vi "cDAQ DDS Set.vi"(5 "common f [Hz]":dbl=1000.0, 6 "ofs [V]":dbl[](array[numeric]), 7 "f [Hz] (empty)":dbl[](array[numeric]), 8 "error in":errorcluster, 9 "ph [rad]":dbl[](array[numeric]), 10 "A [V]":dbl[](array[numeric]), 11 "cDAQ dds":T1={"device"="", "channels"=[], "mclk source"="", "mclk [Hz]"=0.0, "fs [Hz]"=0.0, "block [s]"=0.0, "buf [s]"=0.0, "task"="", "cmd queue"=refnum, "proc ref"=refnum, "smpl clock out"="/cDAQ3/PFI0", "export smpl clock"=FALSE, "DC ofs [V]"=[], "timebase source"="", "timebase mode"=enum."Local", "dither"=enum."Disabled", "dither level"=0.0} {"channels" min=0 step=1}) -> (0 "error out":errorcluster, 3 "cDAQ dds out":T1={"device"="", "channels"=[], "mclk source"="", "mclk [Hz]"=0.0, "fs [Hz]"=0.0, "block [s]"=0.0, "buf [s]"=0.0, "task"="", "cmd queue"=refnum, "proc ref"=refnum, "smpl clock out"="/cDAQ3/PFI0", "export smpl clock"=FALSE, "DC ofs [V]"=[], "timebase source"="", "timebase mode"=enum."Local", "dither"=enum."Disabled", "dither level"=0.0} {"channels" min=0 step=1})   [LabVIEW 2020]
uses:
  cDAQ DDS Session.ctl
  cDAQ DDS Setup.ctl
  cDAQ DDS Timebase Mode.ctl
  cDAQ DDS Dither.ctl
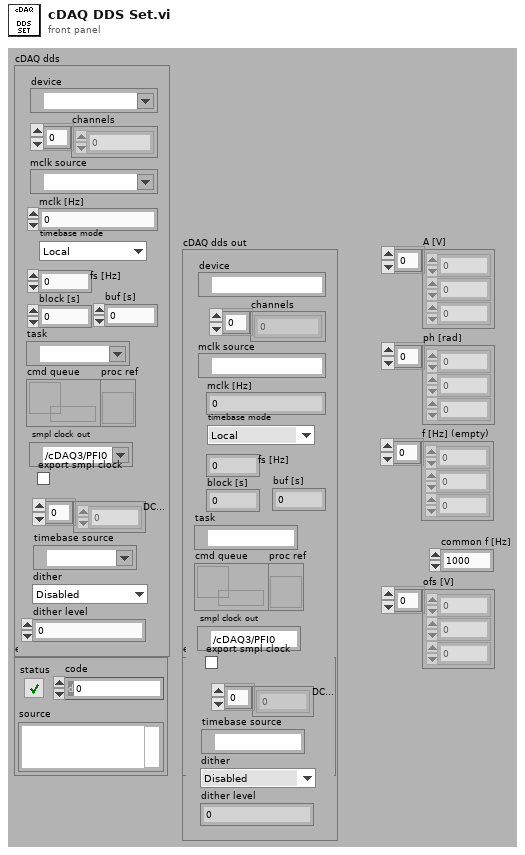
[diagram p1: front panel]
types:
  T1 = typedef "cDAQ DDS Session.ctl" = cluster{"device":tag, "channels":i32[], "mclk source":tag, "mclk [Hz]":dbl, "fs [Hz]":dbl, "block [s]":dbl, "buf [s]":dbl, "task":refnum<k21>, "cmd queue":refnum<queue>, "proc ref":refnum<vi>, "smpl clock out":tag, "export smpl clock":bool, "DC ofs [V]":dbl[], "timebase source":tag, "timebase mode":T2, "dither":T3, "dither level":dbl}
  T2 = typedef "cDAQ DDS Timebase Mode.ctl" = enum16{"Local", "Take from ADC (e.g. NI 9238)", "Other source"}
  T3 = typedef "cDAQ DDS Dither.ctl" = enum16{"Disabled", "Gaussian"}
  T4 = typedef "cDAQ DDS Setup.ctl" = cluster{"A [V]":dbl[], "ph [rad]":dbl[], "f [Hz]":dbl[], "stop":bool, "ofs [V]":dbl[]}
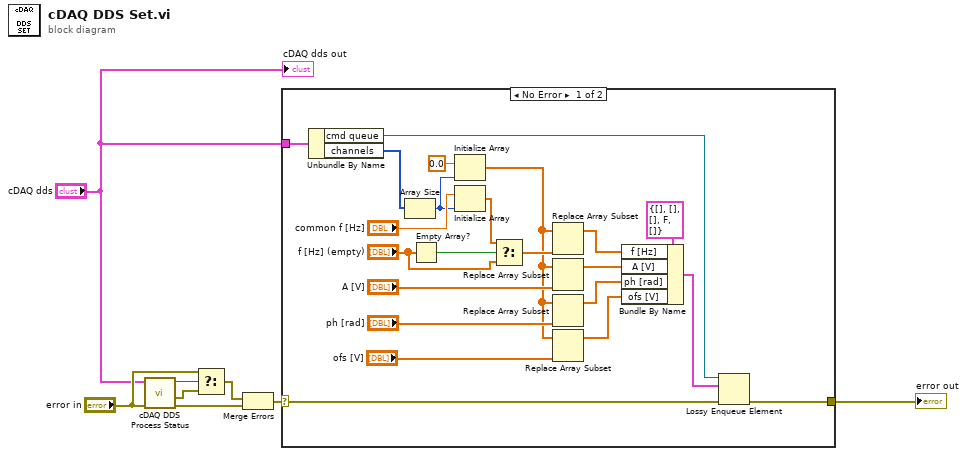
[diagram p0: block diagram]
diagram:
  n1 = call "cDAQ DDS Process Status.vi"("error in"="error in", "cDAQ dds"="cDAQ dds") -> ("error out"=w4:errorcluster, "sweep error out"=w7:errorcluster, "is running"=w8:bool)  [unwired: 7 in]
  n2 = Select(t="error in", s=w8, f=w7) -> (s? t:f=w5:errorcluster)
  n3 = Merge Errors(w5, w4) -> (w3:errorcluster)
  n4 = case shown="No Error" w3 {
    selector: w3 -> [w21 w31]
    tunnel: "cDAQ dds" -> [w28 _]
    tunnel: [w22 w31] -> w2
    frame No Error {
      n5 = Unbundle By Name(w28) -> ("cmd queue"=w24:refnum<queue>, "channels"=w27:i32[])
      n6 = Array Size(array=w27) -> (size(s)=w19:i32)
      n7 = Empty Array?(array="f [Hz] (empty)") -> (empty?=w30:bool)
      n8 = Initialize Array(0.0 ("element"), w19) -> (w9:dbl[])
      n9 = Initialize Array("common f [Hz]", w19) -> (w26:dbl[])
      n10 = Select(t=w26, s=w30, f="f [Hz] (empty)") -> (s? t:f=w16:dbl[])
      n11 = Replace Array Subset(array=w9, new element=w16) -> (w17:dbl[])  [unwired: 1 in]
      n12 = Replace Array Subset(array=w9, new element="A [V]") -> (w15:dbl[])  [unwired: 1 in]
      n13 = Replace Array Subset(array=w9, new element="ph [rad]") -> (w13:dbl[])  [unwired: 1 in]
      n14 = Replace Array Subset(array=w9, new element="ofs [V]") -> (w11:dbl[])  [unwired: 1 in]
      n15 = Bundle By Name(cluster=T4 {"A [V]"=[], "ph [rad]"=[], "f [Hz]"=[], "stop"=FALSE, "ofs [V]"=[]} ("cDAQ dds setup"), "f [Hz]"=w17, "A [V]"=w15, "ph [rad]"=w13, "ofs [V]"=w11) -> (w23:T4)
      n16 = Lossy Enqueue Element(queue=w24, element=w23, error in (no error)=w21) -> (error out=w22:errorcluster)  [unwired: 3 out]
    }
    frame Error {
    }
  }
  "error out" <- w2
  "cDAQ dds out" <- "cDAQ dds"
